vi "Update Input Polarity All Pins.vi"(6 "Input Polarity Cache in":u16, 8 "error in (no error)":errorcluster, 9 "Input Polarity":u16 format="%.0b", 11 "Chip Address (A2 A1 A0)":T2 max=7) -> (0 "error out":errorcluster, 3 "SPI Command":T1, 4 "Input Polarity Cache out":u16)   [LabVIEW 2014, in "SLSC configuration Shared.lvlib"]
doc: "Sets the input polarity logic state (0 = Same Logic State, 1 = Opposite Logic State) for each pin on the chip."
uses:
  CD/Source/Shared/SLSC configuration Shared.lvlib
  Chip Address.ctl
  SPI Command.ctl
  IOCON BANK 0 Reg Addresses.ctl
panel:
  # "Same Logic State = 0\nOpposite Logic State = 1"
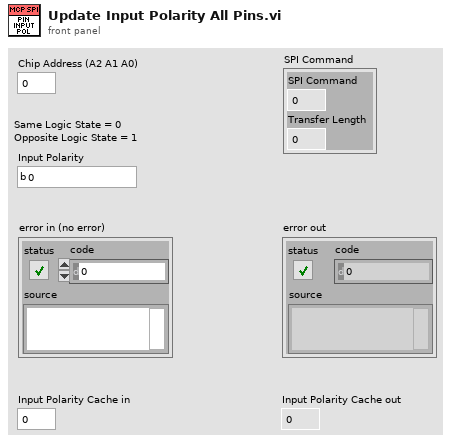
[diagram p1: front panel]
types:
  T1 = typedef "SLSC configuration Shared.lvlib/SPI Command.ctl" = cluster{"SPI Command":u32, "Transfer Length":u8}
  T2 = typedef "SLSC configuration Shared.lvlib/Chip Address.ctl" = u8
  T3 = typedef "SLSC configuration Shared.lvlib/IOCON BANK 0 Reg Addresses.ctl" = enum8{"IODIRA", "IODIRB", "IPOLA", "IPOLB", "GPINTENA", "GPINTENB", "DEFVALA", "DEFVALB", "INTCONA", "INTCONB", "IOCONA", "IOCONB", "GPPUA", "GPPUB", "INTFA", "INTFB", "INTCAPA", "INTCAPB", "GPIOA", "GPIOB", "OLATA", "OLATB"}
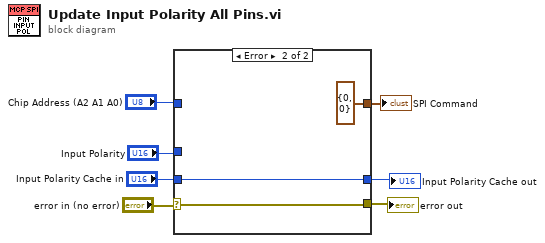
[diagram p0: block diagram]
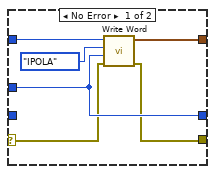
[diagram p2: hidden frame]
diagram:
  n1 = case shown="Error" "error in (no error)" {
    selector: "error in (no error)" -> [w10 w15]
    tunnel: "Chip Address (A2 A1 A0)" -> [w13 _]
    tunnel: [w12 T1 {"SPI Command"=0, "Transfer Length"=0} ("SPI Command")] -> w1
    tunnel: "Input Polarity" -> [w11 _]
    tunnel: "Input Polarity Cache in" -> [_ w16]
    tunnel: [w11 w16] -> w5
    tunnel: [w9 w15] -> w2
    frame No Error {
      n2 = call "Write Word.vi"("error in (no error)"=w10, "Value"=w11, "Reg Address"=IOCON_BANK_0_Reg_Addresses."IPOLA", "Chip Address (A2 A1 A0)"=w13) -> ("error out"=w9:errorcluster, "SPI Command"=w12:T1)  [unwired: 6 in]
    }
    frame Error {
    }
  }
  "Input Polarity Cache out" <- w5
  "error out" <- w2
  "SPI Command" <- w1
